vi "GrowInfo.vi"(1 "XRef":refnum<vi>, 2 "State In":T5) -> (0 "Grow Info":T4)   [LabVIEW 2012, in "Array Size Unbundle.xnode"]
uses:
  Array Size Unbundle.xnode
  State.ctl
  <vilib>/XNodeSupport/XNodeBounds.ctl
  <vilib>/XNodeSupport/XNodeInt.ctl
  <vilib>/XNodeSupport/XNodeBool.ctl
  <vilib>/XNodeSupport/NI_XNodeSupport.lvlib
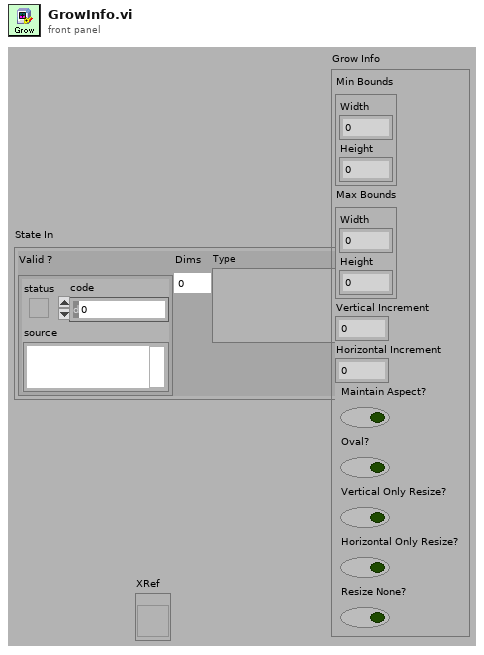
[diagram p1: front panel]
types:
  T1 = typedef "NI_XNodeSupport.lvlib/XNodeBounds.ctl" = cluster{"Width":T2, "Height":T2}
  T2 = typedef "NI_XNodeSupport.lvlib/XNodeInt.ctl" = i32
  T3 = typedef "NI_XNodeSupport.lvlib/XNodeBool.ctl" = bool
  T4 = cluster{"Min Bounds":T1, "Max Bounds":T1, "Vertical Increment":T2, "Horizontal Increment":T2, "Maintain Aspect?":T3, "Oval?":T3, "Vertical Only Resize?":T3, "Horizontal Only Resize?":T3, "Resize None?":T3}
  T5 = typedef "Array Size Unbundle.xnode/State.ctl" = cluster{"Valid ?":errorcluster, "Dims":i32, "Type":variant}
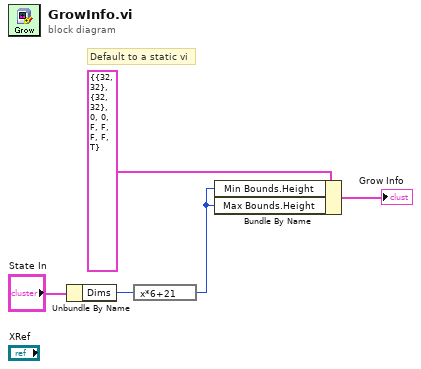
[diagram p0: block diagram]
diagram:
  # "Default to a static vi"
  n1 = Unbundle By Name("State In") -> ("Dims"=w2:i32)
  n2 = expression code="x*6+21"(w2) -> (w1:i32)
  n3 = Bundle By Name(cluster=T4 {"Min Bounds"={"Width"=32, "Height"=32}, "Max Bounds"={"Width"=32, "Height"=32}, "Vertical Increment"=0, "Horizontal Increment"=0, "Maintain Aspect?"=FALSE, "Oval?"=FALSE, "Vertical Only Resize?"=FALSE, "Horizontal Only Resize?"=FALSE, "Resize None?"=TRUE} ("Grow Info"), "Min Bounds.Height"=w1, "Max Bounds.Height"=w1) -> (→"Grow Info":T4)
